vi "setUp.vi"(8 "error in (no error)":errorcluster, 11 "reference in":refnum<class "SLSC EDS System Tests.lvclass">=refnum) -> (0 "error out":errorcluster={"status"=TRUE, "code"=1, "source"="VeriStandTestCase.lvclass:MakePathsAbsoluteWithDefaults.vi<ERR>\nCould not find system definition file"}, 3 "reference out":refnum<class "SLSC EDS System Tests.lvclass">)   [LabVIEW 2019, in "SLSC EDS System Tests.lvclass"]
doc: "setUp runs prior to the test method during test execution. Use this method to initialize any object data required by your tests."
uses:
  SLSC EDS System Tests.lvclass
  <vilib>/addons/_JKI Toolkits/VI Tester/TestCase.llb/TestCase.lvclass
  <vilib>/NI/VeriStand Custom Device Testing Tools/VeriStandTestCase/VeriStandTestCase.lvclass
  C:/Program Files (x86)/National Instruments/LabVIEW 2019/vi.lib/addons/_JKI Toolkits/VI Tester/TestCase.llb/TestCase.lvclass
  C:/Dev/GitHub/niveristand-custom-device-testing-tools/VeriStandTestCase/VeriStandTestCase.lvclass
panel:
  in  "System Definition File":path=path "Assets/Test.nivssdf"
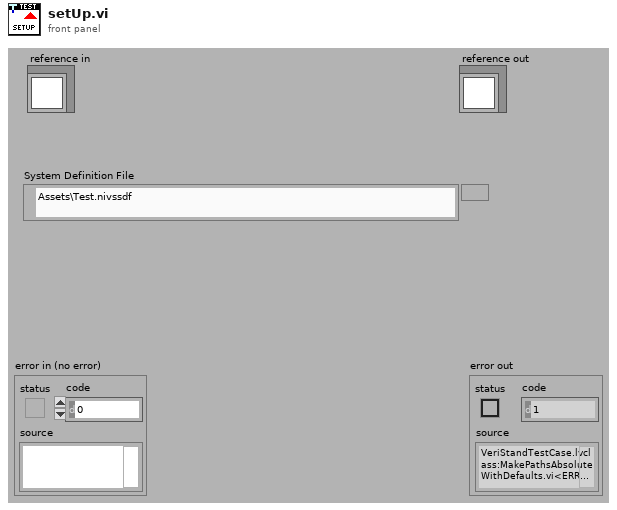
[diagram p1: front panel]
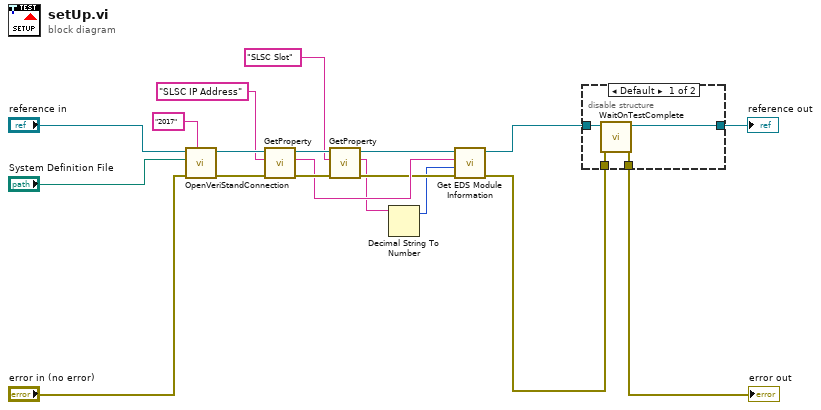
[diagram p0: block diagram]
diagram:
  n1 = call-dynamic "OpenVeriStandConnection.vi"("Minimum VeriStand Version (2016)"="2017" ("Minimum VeriStand Version (2015)"), "error in (no error)"="error in (no error)", "System Definition File"="System Definition File", "VeriStand Test Case in"="reference in") -> ("error out"=w12:errorcluster, "VeriStand Test Case out"=w11:refnum<class "SLSC EDS System Tests.lvclass">)  [unwired: 5 in, 1 out]
  n2 = call <vilib>:"GetProperty.vi"("error in (no error)"=w12, "key"="SLSC IP Address", "VeriStandTestCase in"=w11) -> ("error out"=w9:errorcluster, "value"=w8:string, "VeriStandTestCase out"=w7:refnum<class "SLSC EDS System Tests.lvclass">)  [unwired: 6 in]
  n3 = call <vilib>:"GetProperty.vi"("error in (no error)"=w9, "key"="SLSC Slot", "VeriStandTestCase in"=w7) -> ("error out"=w6:errorcluster, "value"=w3:string, "VeriStandTestCase out"=w5:refnum<class "SLSC EDS System Tests.lvclass">)  [unwired: 6 in]
  n4 = Decimal String To Number(string=w3) -> (offset past number=w2:i32)  [unwired: 2 in, 1 out]
  n5 = call "Get EDS Module Information.vi"("error in (no error)"=w6, "Slot #"=w2, "Chassis IP Address"=w8, "SLSC EDS System Tests in"=w5) -> ("error out"=w16:errorcluster, "SLSC EDS System Tests out"=w17:refnum<class "SLSC EDS System Tests.lvclass">)  [unwired: 6 in]
  n6 = disable-structure shown="Default" {
    disable-tunnel: w16 -> [w23 w24]
    disable-tunnel: [w22 w24] -> w19
    disable-tunnel: [w21 w25] -> w18
    disable-tunnel: w17 -> [w20 w25]
    frame condition #0 (active) {
      n7 = call <vilib>:"WaitOnTestComplete.vi"("error in (no error)"=w23, "TestCase in"=w20) -> ("error out"=w22:errorcluster, "TestCase out"=w21:refnum<class "SLSC EDS System Tests.lvclass">)  [unwired: 8 in]
    }
    frame condition #1 {
    }
  }
  "error out" <- w19
  "reference out" <- w18
